vi "Configure Number of Averages.vi"(8 "error in (no error)":errorcluster {"code" format="%.0x"}, 10 "Number of Averages (16)":i32=16, 11 "VISA Resource Name":refnum<visa-resource-name>) -> (0 "error out":errorcluster {"code" format="%.0x"}, 3 "VISA Resource Name Out":refnum<visa-resource-name>)   [LabVIEW 2010, in "Tektronix TDS 3000 Series.lvlib"]
doc: "Configures the number of waveforms that the oscilloscope acquires and averages. After the oscilloscope acquires as many waveforms as specified, it returns to the Idle state. \n\nNotes:\n\n(1) The tktds3k Configure Acquisition Type VI must be set before calling this VI."
uses:
  <instrlib>/Tektronix TDS 3000 Series/Tektronix TDS 3000 Series.lvlib
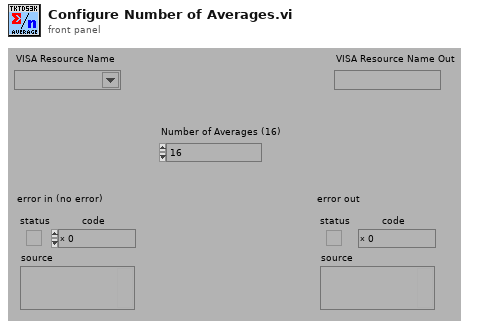
[diagram p1: front panel]
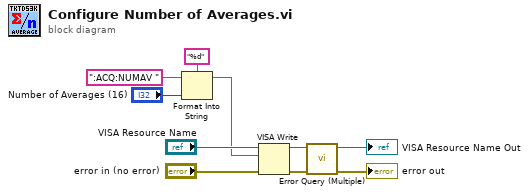
[diagram p0: block diagram]
diagram:
  n1 = Format Into String(format string="%d", initial string=":ACQ:NUMAV ", "Number of Averages (16)") -> (resulting string=w5:string)  [unwired: 1 in, 1 out]
  n2 = VISA Write(VISA resource name="VISA Resource Name", write buffer=w5, error in (no error)="error in (no error)") -> (VISA resource name out=w4:refnum<visa-resource-name>, error out=w3:errorcluster)  [unwired: 1 out]
  n3 = call <instrlib>:"Error Query (Multiple).vi"("error in (no error)"=w3, "VISA Resource Name"=w4) -> ("error out"=→"error out":errorcluster, "VISA Resource Name Out"=→"VISA Resource Name Out":refnum<visa-resource-name>)  [unwired: 6 in, 2 out]
